vi "1_Switch_Case.vi"() -> ()   [LabVIEW 2018]
panel:
  out "Input Valid or Not?":string
  out "Answer":dbl
  in  "Y":dbl
  in  "X":dbl step=1e-07
  in  "Select":T1(ring)
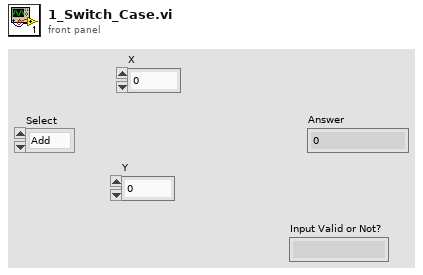
[diagram p1: front panel]
types:
  T1 = enum16{"Add", "Subtract", "Multiply", "Divide", "Average"}
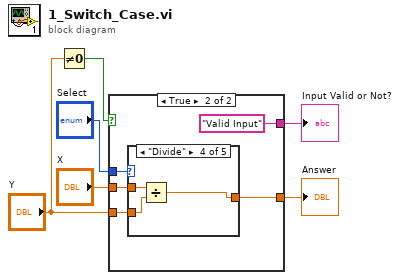
[diagram p0: block diagram]
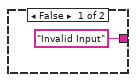
[diagram p2: hidden frame]
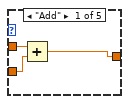
[diagram p3: hidden frame]
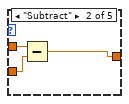
[diagram p4: hidden frame]
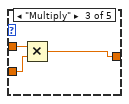
[diagram p5: hidden frame]
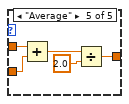
[diagram p6: hidden frame]
diagram:
  n1 = Not Equal To 0?(x="Y") -> (x != 0?=w2:bool)
  n2 = case shown="True" w2 {
    tunnel: "Select" -> [_ w12]
    tunnel: "X" -> [_ w11]
    tunnel: "Y" -> [_ w10]
    tunnel: [_ w9] -> w4
    tunnel: ["Invalid Input" "Valid Input"] -> w3
    frame False {
    }
    frame True {
      n3 = case shown="\"Divide\"" w12 {
        tunnel: w11 -> [w14 w18 w21 w24 w29]
        tunnel: w10 -> [w13 w17 w20 w23 w28]
        tunnel: [w15 w16 w19 w22 w25] -> w9
        frame "Add" {
          n4 = Add(x=w14, y=w13) -> (x+y=w15:dbl)
        }
        frame "Subtract" {
          n5 = Subtract(x=w18, y=w17) -> (x-y=w16:dbl)
        }
        frame "Multiply" {
          n6 = Multiply(x=w21, y=w20) -> (x*y=w19:dbl)
        }
        frame "Divide" {
          n7 = Divide(x=w24, y=w23) -> (x/y=w22:dbl)
        }
        frame "Average" {
          n8 = Add(x=w29, y=w28) -> (x+y=w27:dbl)
          n9 = Divide(x=w27, y=2.0) -> (x/y=w25:dbl)
        }
      }
    }
  }
  "Answer" <- w4
  "Input Valid or Not?" <- w3
